vi "Check Multichassis Sync Support.vi"(8 "error in (no error)":errorcluster, 11 "pxi trigger bus configuration [channel]":T1[](array[typedef])) -> (0 "error out":errorcluster)   [LabVIEW 2019]
uses:
  TypeDefs/PXI Trigger Bus Info.ctl
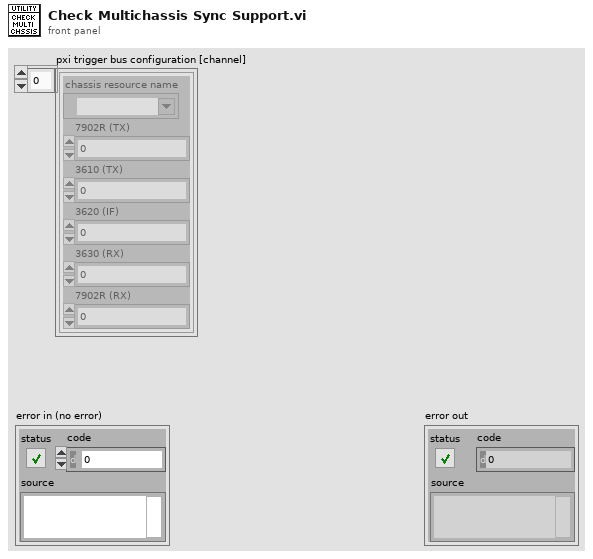
[diagram p1: front panel]
types:
  T1 = typedef "PXI Trigger Bus Info.ctl" = cluster{"chassis resource name":refnum<visa-resource-name>, "7902R (TX)":i16, "3610 (TX)":i16, "3620 (IF)":i16, "3630 (RX)":i16, "7902R (RX)":i16}
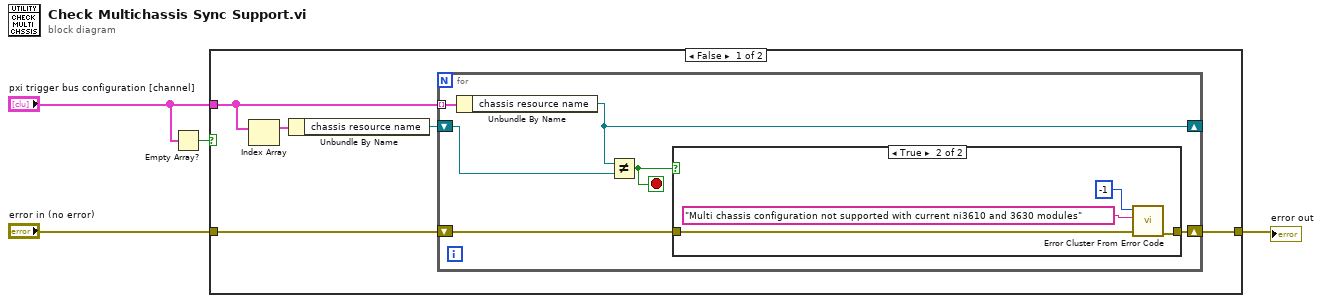
[diagram p0: block diagram]
diagram:
  n1 = Empty Array?(array="pxi trigger bus configuration [channel]") -> (empty?=w1:bool)
  n2 = case shown="False" w1 {
    tunnel: "error in (no error)" -> [w9 w21]
    tunnel: [w8 w21] -> w3
    tunnel: "pxi trigger bus configuration [channel]" -> [w7 _]
    frame False {
      n3 = Index Array(array=w7) -> (element=w5:T1)  [unwired: 1 in]
      n4 = Unbundle By Name(w5) -> ("chassis resource name"=w6:refnum<visa-resource-name>)
      n5 = for {
        tunnel: w7 -> [w15] mode=indexing
        shift-right: [w14] -> _
        shift-left: w6 -> [w13]
        shift-right: [w11] -> w8
        shift-left: w9 -> [w12]
        stop <- w10 stop-if-true
        n6 = Unbundle By Name(w15) -> ("chassis resource name"=w14:refnum<visa-resource-name>)
        n7 = Not Equal?(x=w14, y=w13) -> (x != y?=w10:bool)
        n8 = case shown="True" w10 {
          tunnel: w12 -> [w16 w20]
          tunnel: [w16 w19] -> w11
          frame False {
          }
          frame True {
            n9 = call <vilib>:"Error Cluster From Error Code.vi"("error in (no error)"=w20, "error message (\"\")"="Multi chassis configuration not supported with current ni3610 and 3630 modules" ("error message (\"\")"), "error code (0)"=-1) -> ("error out"=w19:errorcluster)  [unwired: 6 in]
          }
        }
      }
    }
    frame True {
    }
  }
  "error out" <- w3
